vi "Test all Data Types in Variant.vi"() -> ()   [LabVIEW 2015]
uses:
  JSONtext.lvlib
panel:
  out "x = y?":T1
  out "Occurence valid":bool
  out "error out":errorcluster
  out "Queue refun Valid":bool
  out "<JSON>":string
  out "subVariant":variant
  out "Variant out":variant
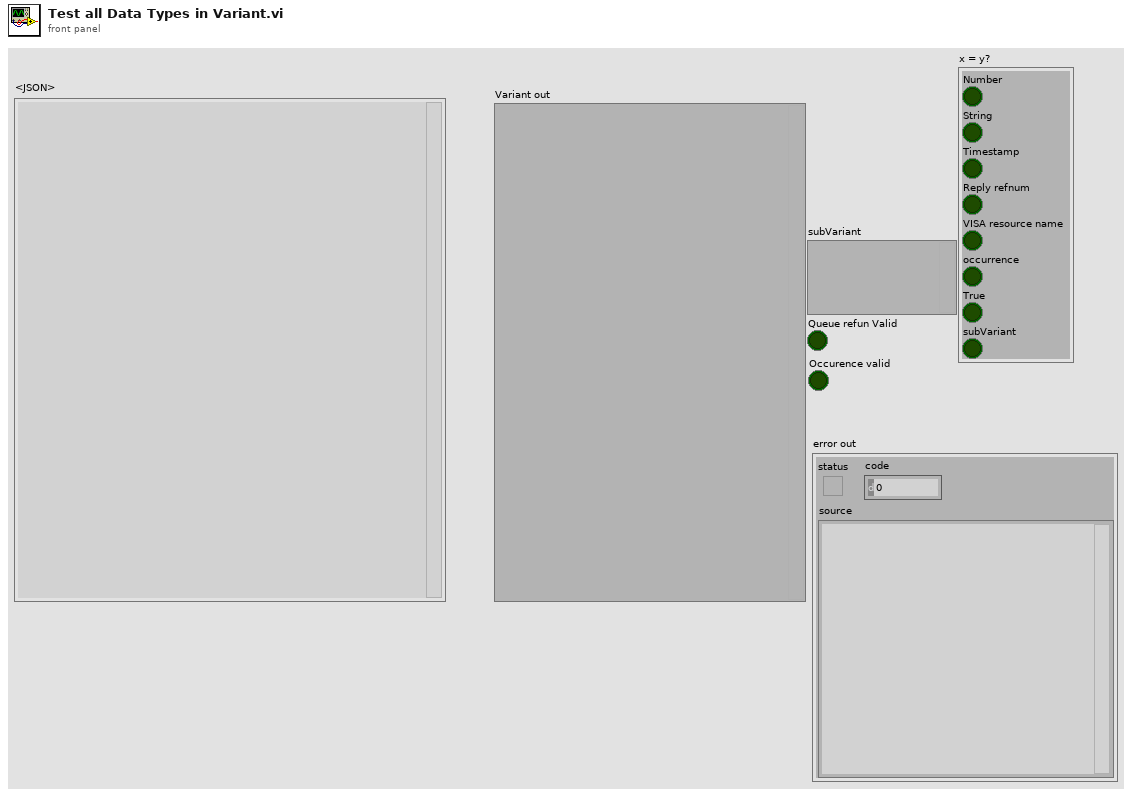
[diagram p1: front panel]
types:
  T1 = cluster{"Number":bool, "String":bool, "Timestamp":bool, "Reply refnum":bool, "VISA resource name":bool, "occurrence":bool, "True":bool, "subVariant":bool}
  T2 = cluster{"Number":i32, "String":string, "Timestamp":timestamp, "Reply refnum":refnum<queue>, "VISA resource name":refnum<visa-resource-name>, "occurrence":refnum<k4>, "True":bool, "subVariant":variant}
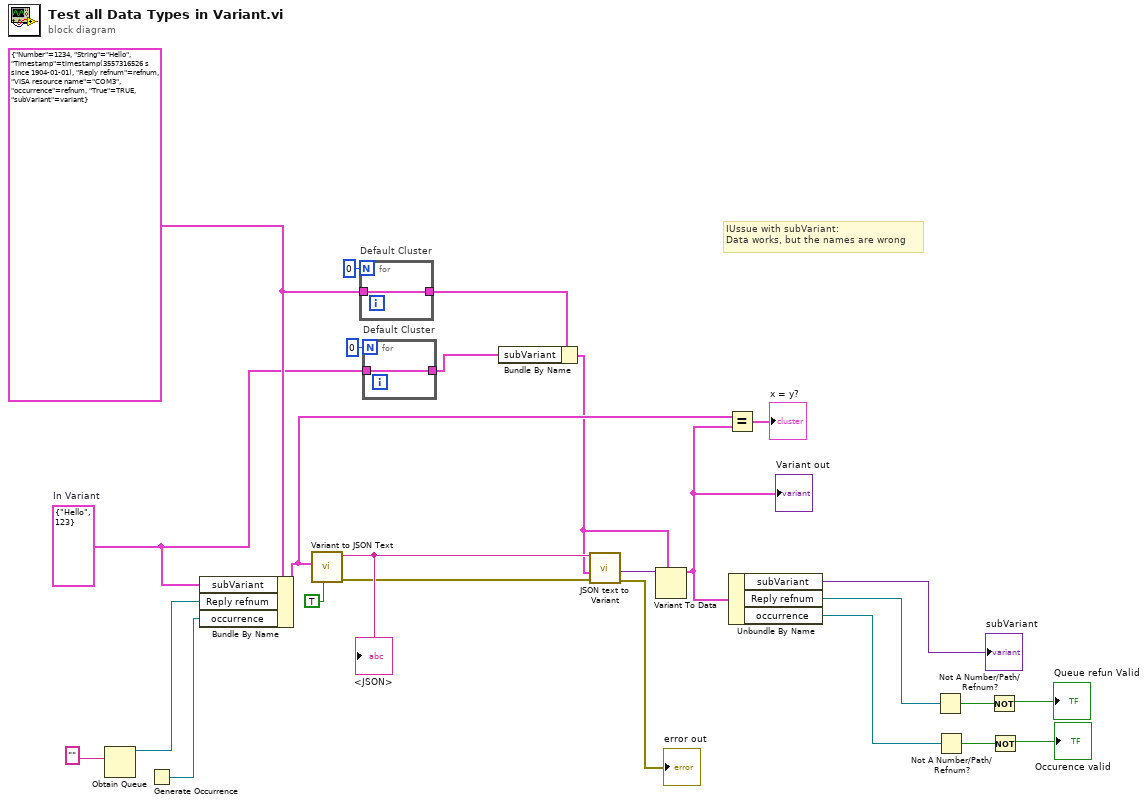
[diagram p0: block diagram]
diagram:
  w4 = cluster{"AAA":string, "123":i32} {"AAA"="Hello", "123"=123}  # In Variant
  w10 = T2 {"Number"=1234, "String"="Hello", "Timestamp"=timestamp(3557316526.864 s since 1904-01-01), "Reply refnum"=refnum, "VISA resource name"="COM3", "occurrence"=refnum, "True"=TRUE, "subVariant"=variant}
  # "IUssue with subVariant:\nData works, but the names are wrong"
  n1 = Obtain Queue(element data type="") -> (queue out=w22:refnum<queue>)  [unwired: 4 in, 2 out]
  n2 = Generate Occurrence() -> (w15:refnum<k4>)
  n3 = Bundle By Name(cluster=w10, "subVariant"=w4, "Reply refnum"=w22, "occurrence"=w15) -> (w11:T2)
  n4 = call "Variant to JSON Text.vi"("Pretty Print?"=TRUE, "Variant"=w11) -> ("error out"=w16:errorcluster, "<JSON>"=w25:string)  [unwired: 7 in, 1 out]
  "<JSON>" <- w25
  n5 = for "Default Cluster" {
    N: 0 -> [_]
    tunnel: w10 -> [w26]
    tunnel: [w26] -> w9
  }
  n6 = for "Default Cluster" {
    N: 0 -> [_]
    tunnel: w4 -> [w27]
    tunnel: [w27] -> w5
  }
  n7 = Bundle By Name(cluster=w9, "subVariant"=w5) -> (w7:T2)
  n8 = call "JSON text to Variant.vi"("error in (no error)"=w16, "Data Type"=w7, "JSON"=w25) -> ("error out"=→"error out":errorcluster, "Variant out"=w3:variant)  [unwired: 7 in]
  n9 = Variant To Data(type=w7, Variant=w3) -> (data=w2:T2)  [unwired: 1 in, 1 out]
  "Variant out" <- w2
  n10 = Equal?(x=w11, y=w2) -> (x = y?=→"x = y?":T1)
  n11 = Unbundle By Name(w2) -> ("subVariant"=→"subVariant":variant, "Reply refnum"=w20:refnum<queue>, "occurrence"=w12:refnum<k4>)
  n12 = Not A Number/Path/Refnum?(number/path/refnum=w20) -> (NaN/Path/Refnum?=w19:bool)
  n13 = Not A Number/Path/Refnum?(number/path/refnum=w12) -> (NaN/Path/Refnum?=w13:bool)
  n14 = Not(x=w19) -> (.not. x?=→"Queue refun Valid":bool)
  n15 = Not(x=w13) -> (.not. x?=→"Occurence valid":bool)
